vi "Initialize-object.vi"(8 "error in (no error)":errorcluster, 9 "Panes settings":T1[](array[typedef]), 10 "VI Reference":refnum<vi>) -> (0 "error out":errorcluster, 3 "Panes out":T5)   [LabVIEW 2013, in "CameraVision.lvlib" / "CV-Panes.lvclass"]
uses:
  CV-Panes.lvclass
  Object-reference.ctl
  Pane-settings.ctl
  Pane-names.ctl
  Splitter-settings.ctl
  Splitter-names.ctl
  CV-Panes.lvclass/CV-Panes.ctl
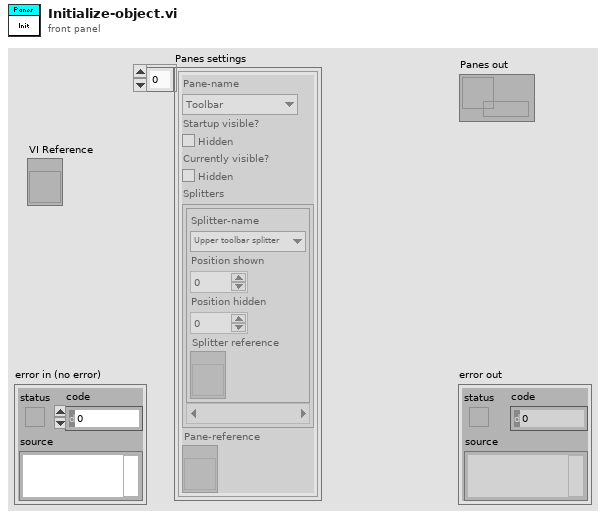
[diagram p1: front panel]
types:
  T1 = typedef "CameraVision.lvlib/CV-Panes.lvclass/Pane-settings.ctl" = cluster{"Pane-name":T2, "Startup visible?":bool, "Currently visible?":bool, "Splitters":T3[], "Pane-reference":refnum<vi>}
  T2 = typedef "CameraVision.lvlib/CV-Panes.lvclass/Pane-names.ctl" = enum16{"Toolbar", "Help bar", "Toolbar lower border", "Settings", "Displays", "Status bar upper border", "General state bar", "Information bar"}
  T3 = typedef "CameraVision.lvlib/CV-Panes.lvclass/Splitter-settings.ctl" = cluster{"Splitter-name":T4, "Position shown":i32, "Position hidden":i32, "Splitter reference":refnum<vi>}
  T4 = typedef "CameraVision.lvlib/CV-Panes.lvclass/Splitter-names.ctl" = enum16{"Upper toolbar splitter", "Help bar splitter", "Lower toolbar splitter", "Upper status bar splitter", "Lower status bar splitter", "Splitter", "Settings splitter"}
  T5 = typedef "CameraVision.lvlib/CV-Panes.lvclass/Object-reference.ctl" = refnum<data-value>
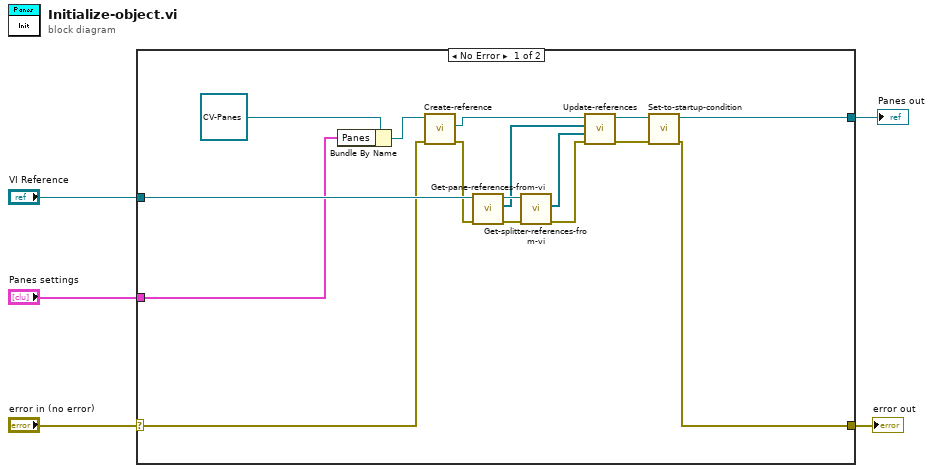
[diagram p0: block diagram]
diagram:
  n1 = case shown="No Error" "error in (no error)" {
    selector: "error in (no error)" -> [w9 w22]
    tunnel: [w8 w22] -> w4
    tunnel: [w7 _] -> w3
    tunnel: "VI Reference" -> [w20 _]
    tunnel: "Panes settings" -> [w6 _]
    frame No Error {
      n2 = Bundle By Name(cluster=refnum<class "CV-Panes.lvclass"> refnum ("Panes.lvclass"), "Panes"=w6) -> (w18:refnum<class "CV-Panes.lvclass">)
      n3 = call "Create-reference.vi"("error in (no error)"=w9, "Panes in"=w18) -> ("error out"=w16:errorcluster, "Panes reference"=w12:T5)  [unwired: 7 in, 1 out]
      n4 = call "Get-pane-references-from-vi.vi"("error in (no error)"=w16, "VI Reference"=w20) -> ("error out"=w15:errorcluster, "Sorted pane references"=w14:refnum<vi>[], "VI Reference out"=w19:refnum<vi>)  [unwired: 7 in]
      n5 = call "Get-splitter-references-from-vi.vi"("error in (no error)"=w15, "VI Reference"=w19) -> ("error out"=w17:errorcluster, "Sorted splitter references"=w13:refnum<vi>[])  [unwired: 7 in, 1 out]
      n6 = call "Update-references.vi"("error in (no error)"=w17, "Sorted splitter references"=w13, "Sorted pane references"=w14, "Panes in"=w12) -> ("error out"=w10:errorcluster, "Panes out"=w11:T5)  [unwired: 6 in]
      n7 = call "Set-to-startup-condition.vi"("error in (no error)"=w10, "Panes in"=w11) -> ("error out"=w8:errorcluster, "Panes out"=w7:T5)  [unwired: 8 in]
    }
    frame Error {
    }
  }
  "error out" <- w4
  "Panes out" <- w3
